vi "Initialize Panel.vi"(8 "error in (no error)":errorcluster, 11 "vi reference in":refnum<vi>) -> (0 "error out":errorcluster, 2 "initial window state":T1(ring), 3 "vi reference out":refnum<vi>)   [LabVIEW 2019, in "Service Template.lvlib"]
uses:
  Service Template.lvlib
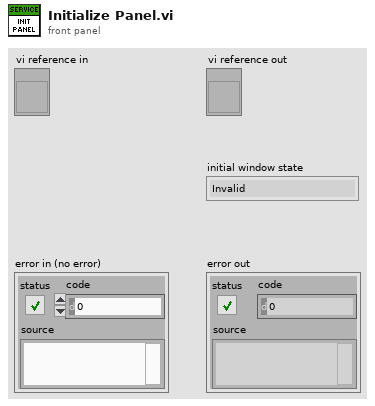
[diagram p1: front panel]
types:
  T1 = enum32{"Invalid", "Standard", "Closed", "Hidden", "Minimized", "Maximized"}
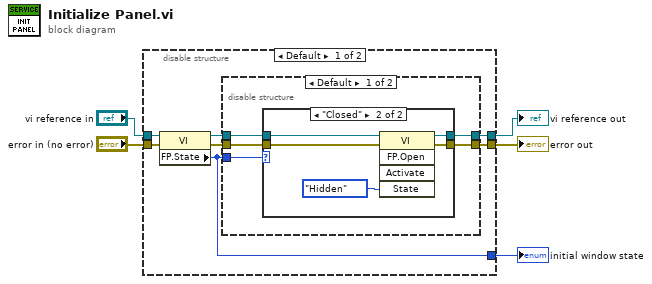
[diagram p0: block diagram]
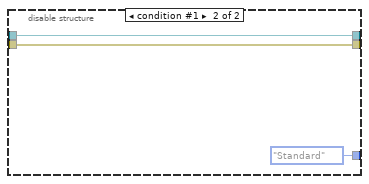
[diagram p4: hidden frame]
diagram:
  n1 = disable-structure shown="Default" {
    disable-tunnel: "vi reference in" -> [w12 w28]
    disable-tunnel: [w9 T1."Standard" ("FP.State")] -> w4
    disable-tunnel: "error in (no error)" -> [w8 w29]
    disable-tunnel: [w7 w28] -> w2
    disable-tunnel: [w6 w29] -> w1
    frame condition #0 (active) {
      n2 = property class="VI"(reference=w12, error in=w8) -> (reference out=w11:refnum<vi>, error out=w10:errorcluster, "FP.State"=w9:T1)
      n3 = disable-structure shown="Default" {
        disable-tunnel: w11 -> [w17 w26]
        disable-tunnel: w10 -> [w16 w25]
        disable-tunnel: w9 -> [w13 _]
        disable-tunnel: [w15 w25] -> w6
        disable-tunnel: [w14 w26] -> w7
        frame condition #0 (active) {
          n4 = case shown="\"Closed\"" w13 {
            tunnel: w17 -> [w19 w23]
            tunnel: w16 -> [w18 w22]
            tunnel: [w18 w21] -> w15
            tunnel: [w19 w20] -> w14
            frame Default {
            }
            frame "Closed" {
              n5 = invoke class="VI" method="FP.Open"(reference=w23, error in=w22, "State"=T1."Hidden") -> (reference out=w20:refnum<vi>, error out=w21:errorcluster)  [unwired: 2 in, 3 out]
            }
          }
        }
        frame condition #1 {
        }
      }
    }
    frame condition #1 {
    }
  }
  "vi reference out" <- w2
  "error out" <- w1
  "initial window state" <- w4
